vi "Fetch Class Methods Info.vi"(5 "Parser Settings":T9, 8 "Error in":errorcluster caption="Error in (no error)", 11 "LVClassLibrary":refnum<vi>) -> (0 "Error out":errorcluster, 2 "Methods":T1[](array[typedef]))   [LabVIEW 2023, in "VIDoc Parsing.lvlib"]
uses:
  VIDoc Parsing.lvlib
  Settings/Parser Settings/Parser Settings Cluster.ctl
  Settings/Parser Settings/Draw Controls Cluster.ctl
  Settings/Parser Settings/Draw Option Enum.ctl
  TypeDefs/Method Spec Cluster.ctl
  TypeDefs/VI Type Extended Enum.ctl
  <vilib>/picture/picture.llb/imagedata.ctl
  TypeDefs/Class Dispatch Type Enum.ctl
  TypeDefs/Controls Info Cluster.ctl
  <vilib>/Utility/miscctls.llb/LVKeyTypeDef.ctl
  <vilib>/Utility/miscctls.llb/LVPointTypeDef.ctl
  Structure Reporter/Tree Cluster.ctl
  Structure Reporter/Structure Reporter.lvlib
  Settings/Parser Settings/Parser Settings.lvclass
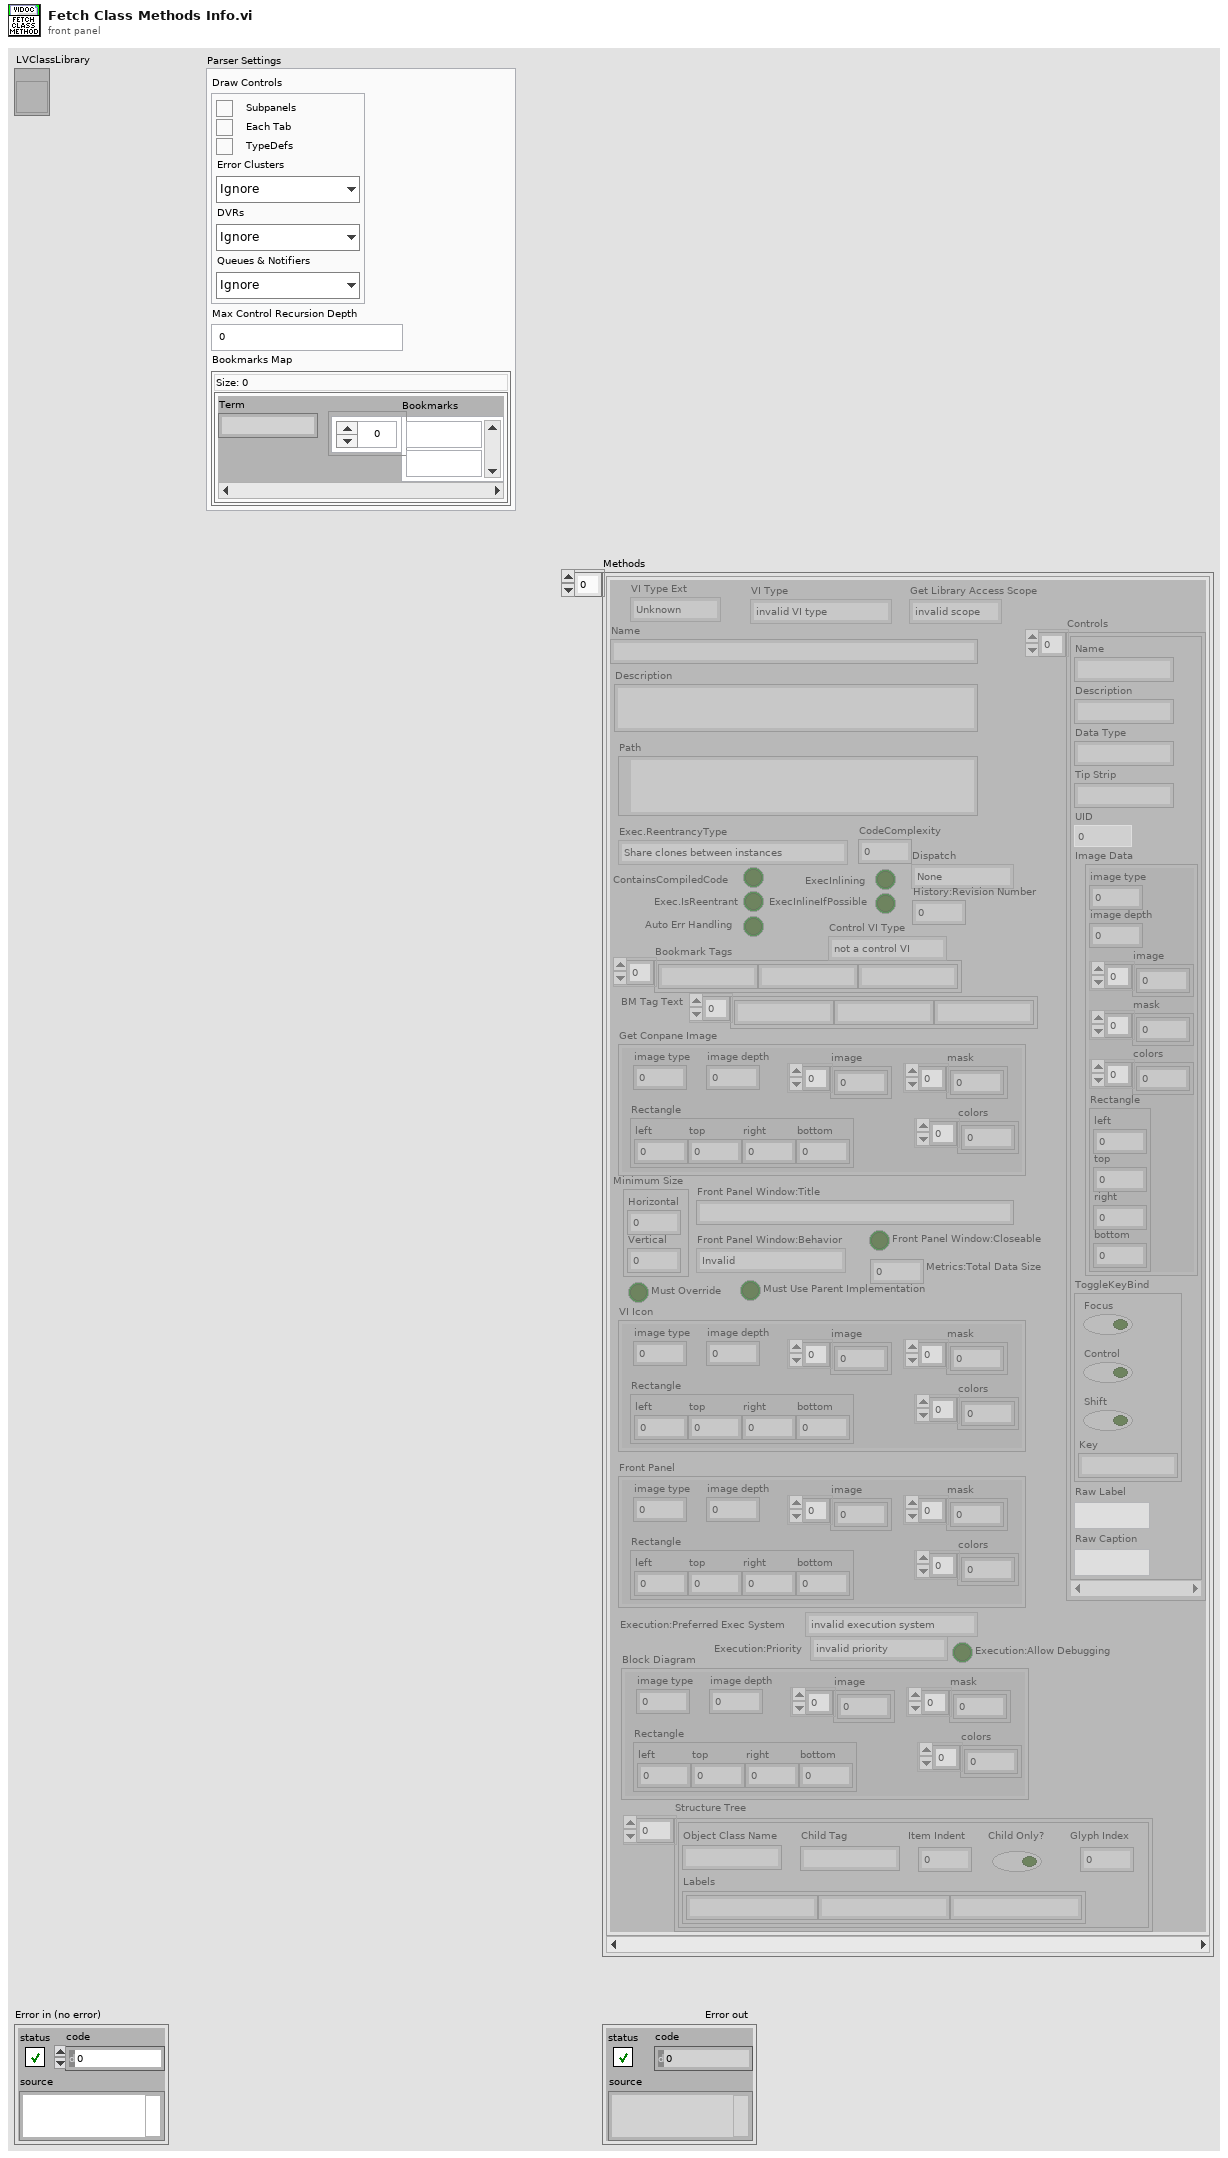
[diagram p1: front panel]
types:
  T1 = typedef "VIDoc Parsing.lvlib/Method Spec Cluster.ctl" = cluster{"VI Type Ext":T2, "Name":string, "Path":path, "Get Conpane Image":T3, "Description":string, "Get Library Access Scope":enum32{"invalid scope", "public", "private", "protected", "community"}, "Dispatch":T4, "ContainsCompiledCode":bool, "Exec.IsReentrant":bool, "Exec.ReentrancyType":enum16{"Share clones between instances", "Preallocate clone for each instance"}, "ExecInlining":bool, "ExecInlineIfPossible":bool, "Auto Err Handling":bool, "CodeComplexity":sgl, "Bookmark Tags":string[], "Control VI Type":enum32{"not a control VI", "control", "typedef", "strict typedef"}, "Controls":T5[], "VI Type":enum32{"invalid VI type", "Standard VI", "Control VI", "Global VI", "Polymorphic VI", "Configuration VI", "SubSystem", "Facade VI", "Method VI", "Statechart Diagram VI"}, "Minimum Size":T7, "Front Panel Window:Title":string, "Front Panel Window:Behavior":enum32{"Invalid", "Default", "Floating", "Floating/Auto-Hide", "Modal"}, "Front Panel Window:Closeable":bool, "Must Override":bool, "Must Use Parent Implementation":bool, "VI Icon":T3, "Front Panel":T3, "History:Revision Number":u32, "Metrics:Total Data Size":u32, "Execution:Allow Debugging":bool, "Execution:Preferred Exec System":enum32{"invalid execution system", "user interface", "standard", "instrument i/o", "data acquisition", "other 1", "other 2", "same as caller"}, "Execution:Priority":enum32{"invalid priority", "background priority", "normal priority", "above normal priority", "high priority", "time critical priority", "subroutine"}, "BM Tag Text":string[], "Block Diagram":T3, "Structure Tree":T8[]}
  T2 = typedef "VIDoc Parsing.lvlib/VI Type Extended Enum.ctl" = enum16{"Unknown", "Class Method", "Class Accessor Get", "Class Accessor Set", "Class Control", "Library Method", "Library Control", "VI", "Control"}
  T3 = typedef "imagedata.ctl" = cluster{"image type":i32, "image depth":i32, "image":u8[], "mask":u8[], "colors":u32[], "Rectangle":cluster{"left":i16, "top":i16, "right":i16, "bottom":i16}}
  T4 = typedef "VIDoc Parsing.lvlib/Class Dispatch Type Enum.ctl" = enum16{"None", "Static", "Dynamic"}
  T5 = typedef "VIDoc Parsing.lvlib/Controls Info Cluster.ctl" = cluster{"Name":string, "Description":string, "Data Type":string, "Tip Strip":string, "UID":i32, "Image Data":T3, "ToggleKeyBind":T6, "Raw Label":string, "Raw Caption":string}
  T6 = typedef "LVKeyTypeDef.ctl" = cluster{"Focus":bool, "Control":bool, "Shift":bool, "Key":string}
  T7 = typedef "LVPointTypeDef.ctl" = cluster{"Horizontal":i16, "Vertical":i16}
  T8 = typedef "VIDoc Parsing.lvlib/Structure Reporter.lvlib/Tree Cluster.ctl" = cluster{"Object Class Name":string, "Labels":string[], "Child Tag":string, "Item Indent":i32, "Child Only?":bool, "Glyph Index":i32}
  T9 = typedef "VIDoc Parsing.lvlib/Parser Settings.lvclass/Parser Settings Cluster.ctl" = cluster{"Draw Controls":T10, "Max Control Recursion Depth":i32, "Bookmarks Map":map{string, string[]}}
  T10 = typedef "VIDoc Parsing.lvlib/Parser Settings.lvclass/Draw Controls Cluster.ctl" = cluster{"Subpanels":bool, "Tabs":bool, "TypeDefs":bool, "Error Clusters":T11, "DVRs":T11, "Queues & Notifiers":T11}
  T11 = typedef "VIDoc Parsing.lvlib/Parser Settings.lvclass/Draw Option Enum.ctl" = enum16{"Ignore", "Draw", "Draw + Contents"}
  T12 = enum32{"invalid VI type", "Standard VI", "Control VI", "Global VI", "Polymorphic VI", "Configuration VI", "SubSystem", "Facade VI", "Method VI", "Statechart Diagram VI"}
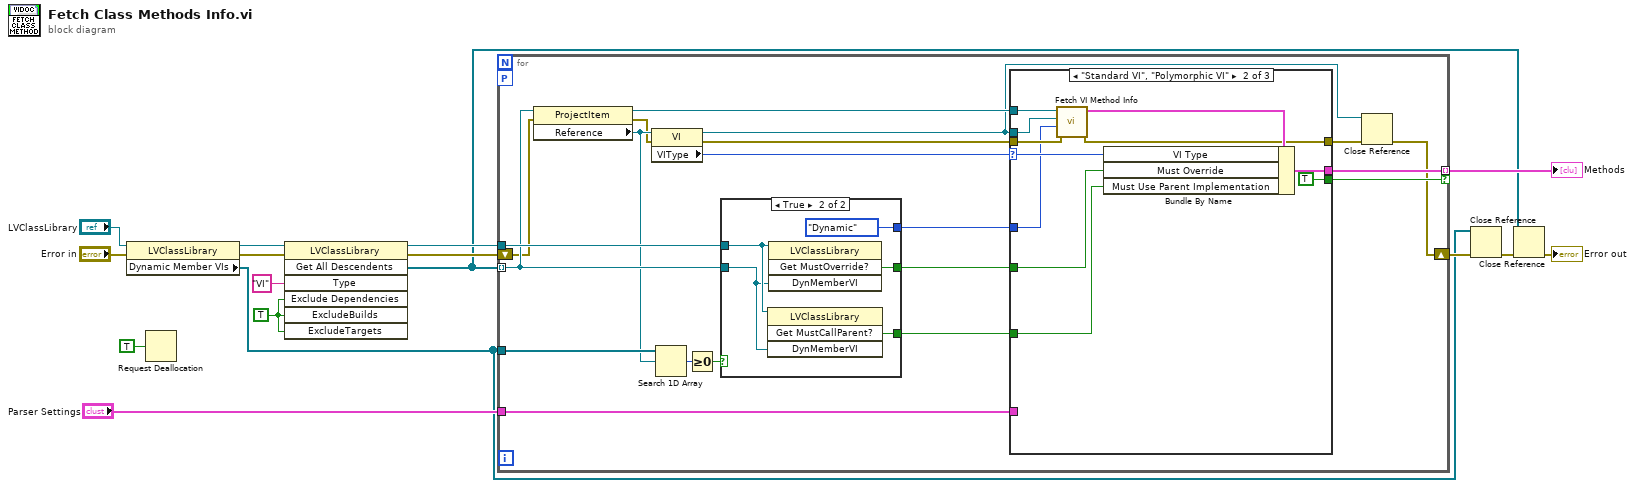
[diagram p0: block diagram]
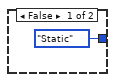
[diagram p2: hidden frame]
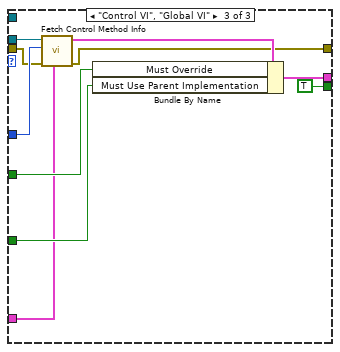
[diagram p4: hidden frame]
diagram:
  w10 = TRUE ("ExcludeDependencies")
  n1 = property class="LVClassLibrary"(reference="LVClassLibrary", error in="Error in") -> (reference out=w13:refnum<vi>, error out=w11:errorcluster, "Dynamic Member VIs"=w4:refnum<vi>[])
  n2 = Request Deallocation(TRUE ("flag")) -> ()
  n3 = invoke class="LVClassLibrary" method="Get All Descendents"(reference=w13, error in=w11, "Type"="VI", "Exclude Dependencies"=w10, "ExcludeBuilds"=w10, "ExcludeTargets"=w10) -> (reference out=w9:refnum<vi>, error out=w7:errorcluster, "All Descendents"=w1:refnum<vi>[])  [unwired: 1 in, 4 out]
  n4 = for {
    tunnel: w4 -> [w29]
    tunnel: [w35] -> w8 mode=indexing if=w34
    tunnel: w9 -> [w33]
    tunnel: w1 -> [w28] mode=indexing
    shift-right: [w18] -> w5
    shift-left: w7 -> [w23]
    tunnel: "Parser Settings" -> [w19]
    workers-P: _ -> [_]
    n5 = property class="ProjectItem"(reference=w28, error in=w23) -> (reference out=w32:refnum<vi>, error out=w22:errorcluster, "Reference"=w27:refnum<vi>)
    n6 = property class="VI"(reference=w27, error in=w22) -> (reference out=w17:refnum<vi>, error out=w21:errorcluster, "VIType"=w36:T12)
    n7 = Search 1D Array(1D array=w29, element=w27) -> (index of element=w26:i32)  [unwired: 1 in]
    n8 = Greater Or Equal To 0?(x=w26) -> (x >= 0?=w25:bool)
    n9 = case shown="True" w25 {
      tunnel: w33 -> [_ w42]
      tunnel: w28 -> [_ w41]
      tunnel: [_ w40] -> w30
      tunnel: [_ w39] -> w31
      tunnel: [Class_Dispatch_Type_Enum."Static" Class_Dispatch_Type_Enum."Dynamic"] -> w24
      frame False {
      }
      frame True {
        n10 = invoke class="LVClassLibrary" method="Get MustCallParent?"(reference=w42, "DynMemberVI"=w41) -> ("Get MustCallParent?"=w39:bool)  [unwired: 2 in, 3 out]
        n11 = invoke class="LVClassLibrary" method="Get MustOverride?"(reference=w42, "DynMemberVI"=w41) -> ("GetMustOverride"=w40:bool)  [unwired: 2 in, 3 out]
      }
    }
    n12 = case shown="\"Standard VI\", \"Polymorphic VI\"" w36 {
      selector: w36 -> [_ w53 _]
      tunnel: w17 -> [_ w44 w59]
      tunnel: w24 -> [_ w45 w58]
      tunnel: w32 -> [_ w49 _]
      tunnel: [_ w52 w61] -> w35
      tunnel: [_ TRUE TRUE] -> w34
      tunnel: w30 -> [_ w51 w63]
      tunnel: w31 -> [_ w50 w62]
      tunnel: w21 -> [w43 w47 w57]
      tunnel: [w43 w46 w56] -> w20
      tunnel: w19 -> [_ _ w55]
      frame Default {
      }
      frame "Standard VI", "Polymorphic VI" {
        n13 = call "Fetch VI Method Info.vi"("Error in"=w47, "Dispatch (None)"=w45, "VI Reference"=w44, "VI ProjectItem in"=w49) -> ("Error out"=w46:errorcluster, "Method Spec Cluster"=w48:T1)  [unwired: 6 in]
        n14 = Bundle By Name(cluster=w48, "VI Type"=w53, "Must Override"=w51, "Must Use Parent Implementation"=w50) -> (w52:T1)
      }
      frame "Control VI", "Global VI" {
        n15 = call "Fetch Control Method Info.vi"("Parser Settings"=w55, "Error in"=w57, "Dispatch (None)"=w58, "VI in"=w59) -> ("Error out"=w56:errorcluster, "Method Spec Cluster"=w60:T1)  [unwired: 6 in]
        n16 = Bundle By Name(cluster=w60, "Must Override"=w63, "Must Use Parent Implementation"=w62) -> (w61:T1)
      }
    }
    n17 = Close Reference(reference=w17, error in (no error)=w20) -> (error out=w18:errorcluster)
  }
  "Methods" <- w8
  n18 = Close Reference(reference=w4, error in (no error)=w5) -> (error out=w3:errorcluster)
  n19 = Close Reference(reference=w1, error in (no error)=w3) -> (error out=→"Error out":errorcluster)
